vi "Stop Core.vi"(10 "final error code":i32, 11 "root_actor in":refnum<class "root_actor.lvclass">) -> (3 "root_actor out":refnum<class "root_actor.lvclass">)   [LabVIEW 2025, in "root_actor.lvlib" / "root_actor.lvclass"]
doc: "(<B>Filename</B>: Actor Framework.lvlib:Actor.lvclass:Stop Core.vi)\n\nDefines what the actor does before it stops. Use the <B>final error code</B> input to determine whether the actor shut down in response to an error.\n\nBy default, this method passes the Stop message along to all auto-stop nested actors. A descendant class may override this method to define additional behavior, such as shutting down any processes the actor initiated in its override of the Actor Core method."
uses:
  root_actor.lvclass
  <vilib>/ActorFramework/Actor/Actor.lvclass
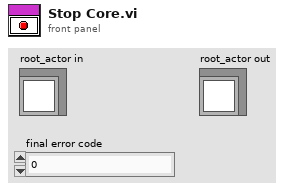
[diagram p1: front panel]
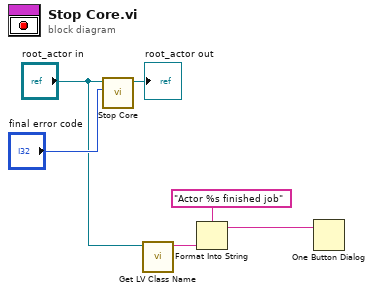
[diagram p0: block diagram]
diagram:
  n1 = call-parent "Stop Core.vi"("final error code"="final error code", "Actor in"="root_actor in") -> ("Actor out"=→"root_actor out":refnum<class "root_actor.lvclass">)  [unwired: 9 in]
  n2 = call <vilib>:"Get LV Class Name.vi"("object"="root_actor in") -> ("class name"=w3:string)  [unwired: 9 in, 1 out]
  n3 = Format Into String(format string="Actor %s finished job", w3) -> (resulting string=w1:string)  [unwired: 2 in, 1 out]
  n4 = One Button Dialog(message=w1) -> ()  [unwired: 1 in, 1 out]
